vi "Modbus Demo TCP Feature.vi"() -> ()   [LabVIEW 2013]
uses:
  C:/Users/User/OneDrive - ITRI/Documents/_Code_LabVIEW/Modbus Demo/DLL/LabVIEW_CSLib.dll
  DLL/LabVIEW_CSLib.dll
  C:/Users/User/OneDrive - ITRI/Documents/_Code_LabVIEW/Modbus Demo/DLL/Modbus.dll
  DLL/Modbus.dll
panel:
  in  "Feature ADDR":u16=25
  out "error out":errorcluster
  out "Device ID":u16
  in  "Port":i32=502
  in  "TCP address":string="192.168.178.2"
  in  "stop":bool
  out "Feature":dbl[][](graph)
  out "Iteration":i32
  in  "DAQ Interval (ms)":u32
  in  "Sample Rate":u16=7812
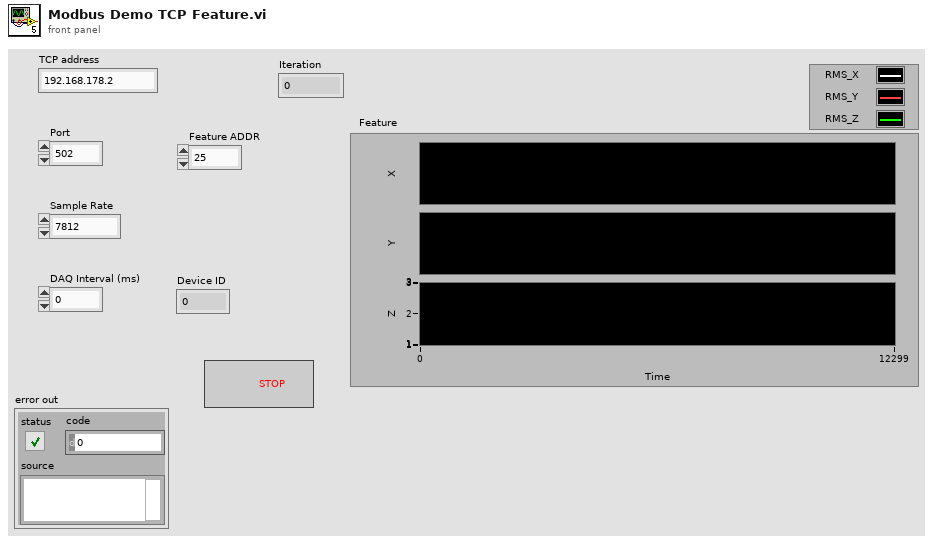
[diagram p1: front panel]
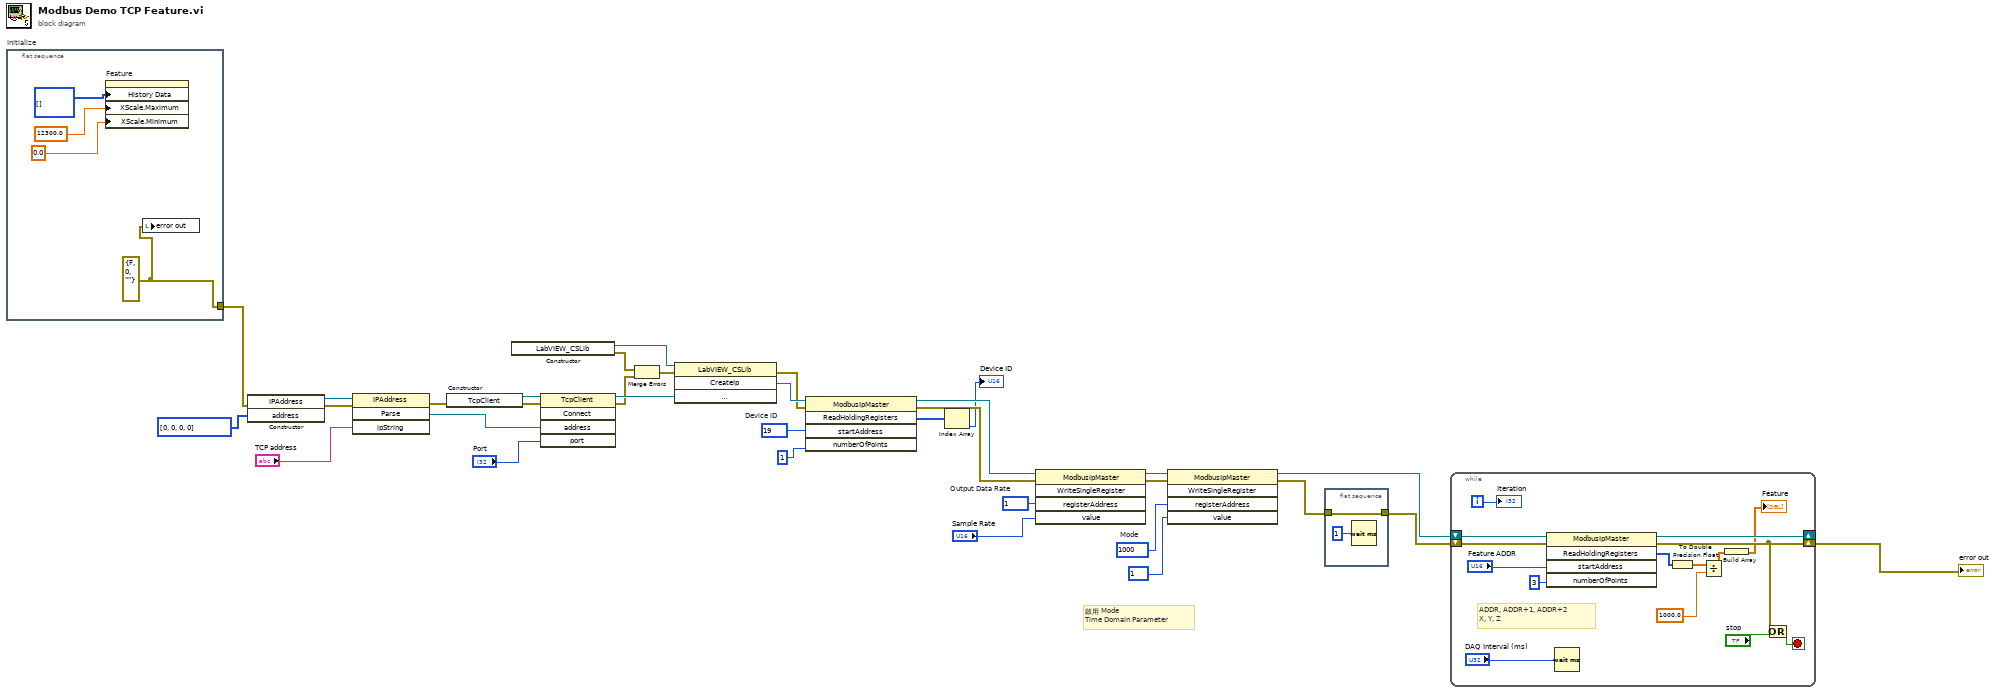
[diagram p0: block diagram]
diagram:
  w6 = u16 1000  # Mode
  w23 = u16 19  # Device ID
  w25 = u16 1  # Output Data Rate
  # "啟用 Mode\nTime Domain Parameter"
  n1 = flat-sequence "Initialize" {
    tunnel: [w34] -> w10
    frame #0 {
      w34 = errorcluster {"status"=FALSE, "code"=0, "source"=""} ("error out")
      n2 = property on="Feature" class="WFChart (strict)"("History Data"=i16[][] [], "XScale.Maximum"=12300.0 ("X Scale.Range:Maximum"), "XScale.Minimum"=0.0 ("X Scale.Range:Minimum")) -> ()  [unwired: 2 in, 2 out]
      n3 = local write "error out"(w34) -> ()
    }
  }
  n4 = constructor class="IPAddress"(error in=w10, "address"=u8[] [0, 0, 0, 0]) -> (reference out=w32:refnum<k24>, error out=w20:errorcluster)  [unwired: 2 in, 2 out]
  n5 = invoke class="IPAddress" method="Parse"(reference=w32, error in=w20, "ipString"="TCP address") -> (error out=w21:errorcluster, "Parse"=w29:refnum<k24>)  [unwired: 1 in, 2 out]
  n6 = constructor class="TcpClient"(error in=w21) -> (reference out=w33:refnum<k24>, error out=w31:errorcluster)  [unwired: 2 in, 1 out]
  n7 = constructor class="LabVIEW_CSLib"() -> (reference out=w16:refnum<k24>, error out=w15:errorcluster)  [unwired: 3 in, 1 out]
  n8 = invoke class="TcpClient" method="Connect"(reference=w33, error in=w31, "address"=w29, "port"="Port") -> (reference out=w27:refnum<k24>, error out=w14:errorcluster)  [unwired: 1 in, 3 out]
  n9 = Merge Errors(w15, w14) -> (w13:errorcluster)
  n10 = invoke class="LabVIEW_CSLib" method="CreateIp"(reference=w16, error in=w13, "tcpClient"=w27) -> (error out=w18:errorcluster, "CreateIp"=w22:refnum<k24>)  [unwired: 1 in, 2 out]
  n11 = invoke class="ModbusIpMaster" method="ReadHoldingRegisters"(reference=w22, error in=w18, "startAddress"=w23, "numberOfPoints"=u16 1) -> (reference out=w19:refnum<k24>, error out=w17:errorcluster, "ReadHoldingRegisters"=w12:u16[])  [unwired: 1 in, 2 out]
  n12 = Index Array(array=w12) -> (element=→"Device ID":u16)  [unwired: 1 in]
  n13 = invoke class="ModbusIpMaster" method="WriteSingleRegister"(reference=w19, error in=w17, "registerAddress"=w25, "value"="Sample Rate") -> (reference out=w4:refnum<k24>, error out=w3:errorcluster)  [unwired: 1 in, 3 out]
  n14 = invoke class="ModbusIpMaster" method="WriteSingleRegister"(reference=w4, error in=w3, "registerAddress"=w6, "value"=u16 1) -> (reference out=w7:refnum<k24>, error out=w8:errorcluster)  [unwired: 1 in, 3 out]
  n15 = flat-sequence {
    tunnel: w8 -> [w38]
    tunnel: [w38] -> w2
    frame #0 {
      n16 = Wait (ms)(milliseconds to wait=u32 1) -> ()  [unwired: 1 out]
    }
  }
  n17 = while {
    shift-right: [w45] -> w1
    shift-left: w2 -> [w47]
    shift-right: [w46] -> _
    shift-left: w7 -> [w50]
    i -> [w53]
    stop <- w51 stop-if-true
    # "ADDR, ADDR+1, ADDR+2\nX, Y, Z"
    n18 = invoke class="ModbusIpMaster" method="ReadHoldingRegisters"(reference=w50, error in=w47, "startAddress"="Feature ADDR", "numberOfPoints"=u16 3) -> (reference out=w46:refnum<k24>, error out=w45:errorcluster, "ReadHoldingRegisters"=w43:u16[])  [unwired: 1 in, 2 out]
    n19 = Wait (ms)(milliseconds to wait="DAQ Interval (ms)") -> ()  [unwired: 1 out]
    n20 = To Double Precision Float(number=w43) -> (double precision float=w41:dbl[])
    n21 = Divide(x=w41, y=1000.0) -> (x/y=w40:dbl[])
    n22 = Build Array(w40) -> (→"Feature":dbl[][])
    n23 = Or(x=w45, y="stop") -> (x .or. y?=w51:bool)
    "Iteration" <- w53
  }
  "error out" <- w1
